vi "2D tether waveforms.vi"(0 "tether sizes":dbl[][](array[numeric]), 1 "Data period (s)":dbl, 2 "Time Stamp":timestamp, 3 "Forces":waveform(dbl)[](array[waveform])) -> (5 "tethers":waveform(dbl)[](array[waveform]), 6 "output forces":waveform(dbl)[](array[waveform]), 7 "Output Means":T1)   [LabVIEW 2014]
uses:
  <vilib>/Analysis/baseanly.llb/Mean (DBL).vi
  <vilib>/Analysis/NI_AALBase.lvlib
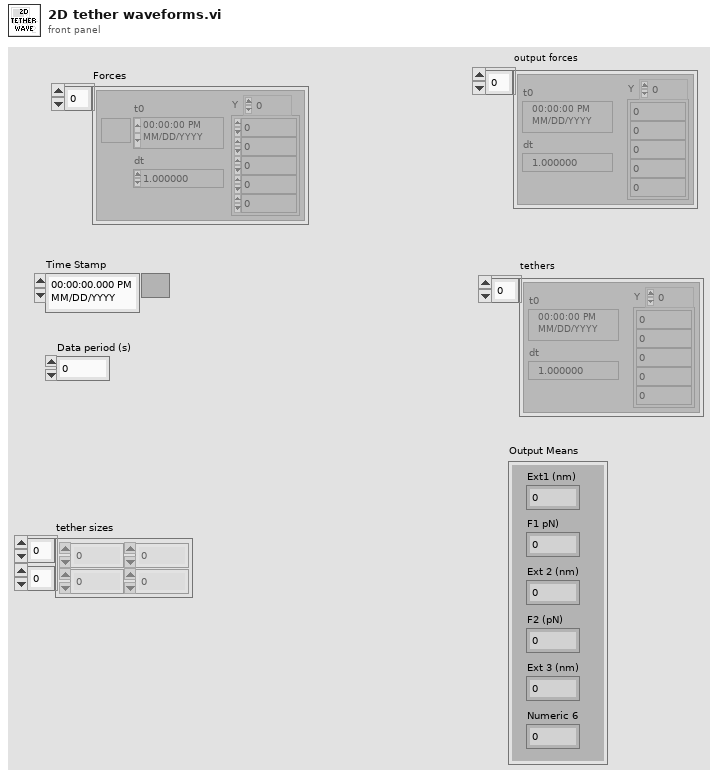
[diagram p1: front panel]
types:
  T1 = cluster{"Ext1 (nm)":dbl, "F1 pN)":dbl, "Ext 2 (nm)":dbl, "F2 (pN)":dbl, "Ext 3 (nm)":dbl, "Numeric 6":dbl}
  T2 = cluster{"[0]":dbl, "[1]":dbl, "[2]":dbl, "[3]":dbl, "[4]":dbl, "[5]":dbl}
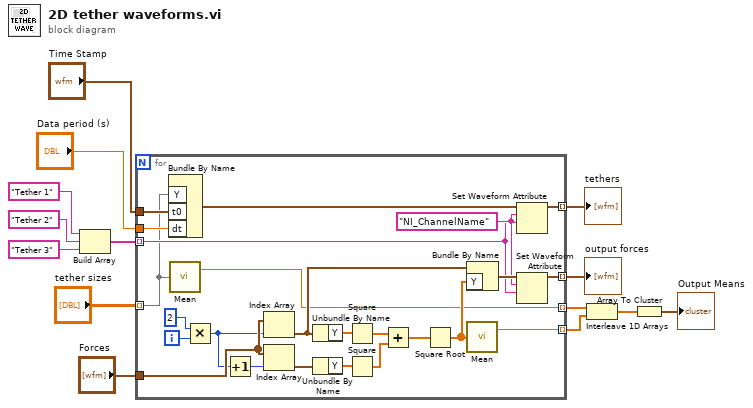
[diagram p0: block diagram]
diagram:
  n1 = Build Array("Tether 1", "Tether 2", "Tether 3") -> (w10:string[])
  n2 = for {
    tunnel: "tether sizes" -> [w18] mode=indexing
    tunnel: [w35] -> w14 mode=indexing
    tunnel: w10 -> [w20] mode=indexing
    tunnel: "Data period (s)" -> [w38]
    tunnel: "Time Stamp" -> [w37]
    tunnel: "Forces" -> [w34]
    tunnel: [w19] -> w5 mode=indexing
    tunnel: [w16] -> w4 mode=indexing
    tunnel: [w15] -> w3 mode=indexing
    i -> [w32]
    w21 = "NI_ChannelName"
    n3 = Bundle By Name("Y"=w18, "t0"=w37, "dt"=w38) -> (w36:waveform(dbl))  [unwired: 1 in]
    n4 = call-poly <vilib>:"Mean.vi"("X"=w18) -> ("mean"=w16:dbl)  [unwired: 1 out]
    n5 = Multiply(x=2, y=w32) -> (x*y=w31:i32)
    n6 = Increment(x=w31) -> (x+1=w30:i32)
    n7 = Index Array(array=w34, index=w31) -> (element=w23:waveform(dbl))
    n8 = Index Array(array=w34, index=w30) -> (element=w29:waveform(dbl))
    n9 = Unbundle By Name(w23) -> ("Y"=w28:dbl[])
    n10 = Unbundle By Name(w29) -> ("Y"=w27:dbl[])
    n11 = Square(x=w28) -> (x^2=w26:dbl[])
    n12 = Square(x=w27) -> (x^2=w25:dbl[])
    n13 = Add(x=w26, y=w25) -> (x+y=w24:dbl[])
    n14 = Square Root(x=w24) -> (sqrt(x)=w17:dbl[])
    n15 = Bundle By Name(cluster=w23, "Y"=w17) -> (w22:waveform(dbl))
    n16 = call-poly <vilib>:"Mean.vi"("X"=w17) -> ("mean"=w15:dbl)  [unwired: 1 out]
    n17 = Set Waveform Attribute(5:w20, 6:w21, 7:w36) -> (3:w35:waveform(dbl))  [unwired: 1 in, 2 out]
    n18 = Set Waveform Attribute(5:w20, 6:w21, 7:w22) -> (3:w19:waveform(dbl))  [unwired: 1 in, 2 out]
  }
  "tethers" <- w14
  "output forces" <- w5
  n19 = Interleave 1D Arrays(w4, w3) -> (w2:dbl[])
  n20 = Array To Cluster(array=w2) -> (cluster=→"Output Means":T2)
